vi "Shot Info Collection.vi"(6 "Vision Target Aligned? in":bool, 7 "Current Angle":dbl, 9 "Shot Type":T1, 10 "Vision Packet":T2, 11 "Shooter Presets":T3={"Batter Shot"={"Left"=0.0, "Right"=0.0, "Angle"=0.0}, "Deep Middle Shot"={"Left"=0.0, "Right"=0.0, "Angle"=0.0}, "Manual Shot"={"Left"=0.0, "Right"=0.0, "Angle"=0.0}, "Left Ticks Per Rotation"=0.0, "Right Ticks Per Rotation"=0.0, "Low Bar Shot"={"Left"=0.0, "Right"=0.0, "Angle"=0.0}, "Shooter RPM Tolerance"=0.0, "IIR Filter Power"=0.0, "Trigger Power"=0.0, "Fire from Load Delay"=0, "Max Angle"=0.0, "Min Angle"=0.0, "Angle PID gains"={"P"=0.0, "I"=0.0, "D"=0.0}, "Angle Output"={"output high"=0.0, "output low"=0.0}, "Shooter Angle Tolerance"=0.0, "Vision Shoot x^2"=0.0, "Vision Shoot x"=0.0, "Offset Angle"=0.0, "High Goal Center Height"=0.0, "Feed Forward Max Accel"=0.0, "Feed Forward Kv"=0.0, "Backwards Trigger"=0.0, "Shot Finish Delay (ms)"=0.0, "Angle Max Current"=0.0, "Angle Current Trip Time"=0.0, "Intake Angle"=0.0, "Vision Shoot c"=0.0, "Reset?"=FALSE, "Servo Release Delay"=0.0, "Servo Idle Angle"=0, "Servo Hold Angle"=0, "Angle Pot x"=0.0, "Angle Pot c"=0.0, "Ignore Angle?"=FALSE, "Manual Output?"=FALSE, "Manual Out"=0.0, "Max RPM"=0.0, "Safty Frist Angle"=0.0, "Intake Danger Height"=0.0, "Angle Pot B"=0, "Angle Pot M"=0.0, "FF Finish RPM"=0.0, "RPM PID Right"={"P"=1.0, "I"=0.01, "D"=0.0, "FF"=0.0}, "RPM PID Left"={"P"=1.0, "I"=0.01, "D"=0.0, "FF"=0.0}, "Backwards RPM"=0.0, "Vision RPM"=0.0, "Run Wheels Backward Delay"=0} {"Angle Output"."output low" format="%.2f"; "Angle Output"."output high" format="%.2f"}) -> (2 "Right Wheel RPM":dbl, 3 "Left Wheel RPM":dbl, 4 "Angle":dbl, 5 "Vision Target Aligned? out":bool)   [LabVIEW 2015]
uses:
  Common Code/Shooter Presets.ctl
  Common Code/Shot Presets.ctl
  Common Code/Goal Vision Packet.ctl
  Common Code/Shot Type.ctl
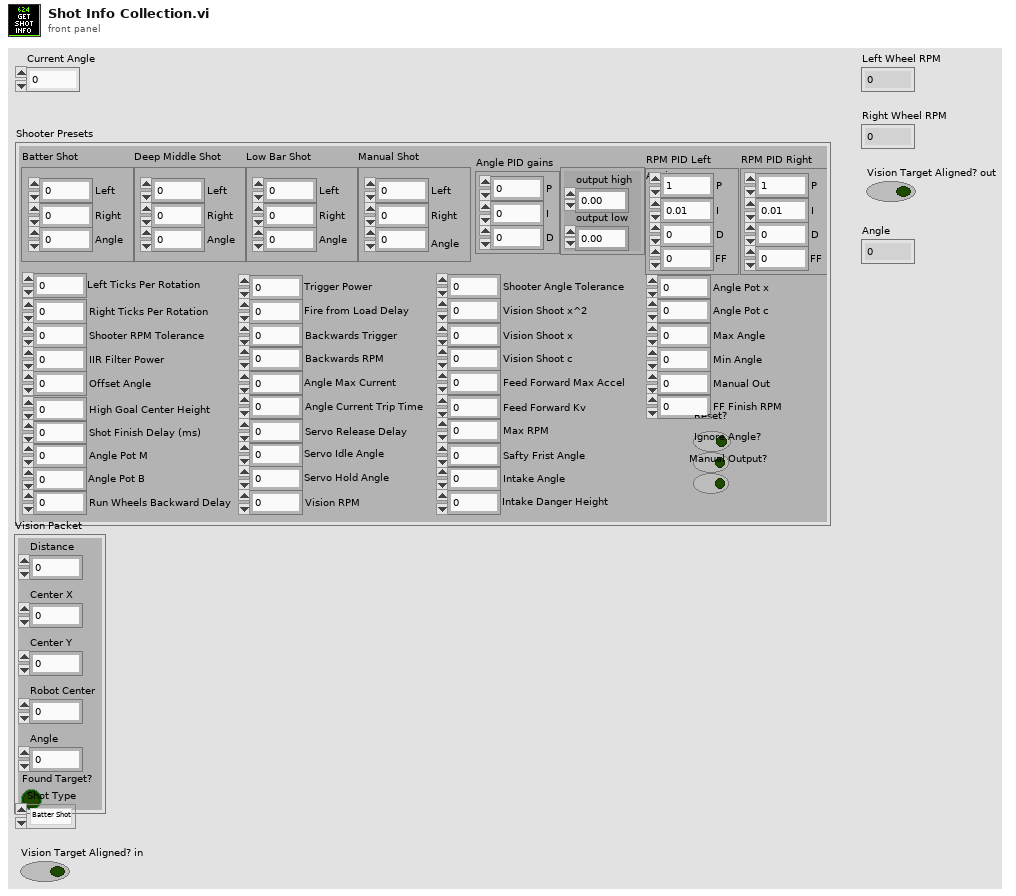
[diagram p1: front panel]
types:
  T1 = typedef "Shot Type.ctl" = enum16{"Batter Shot", "Corner Shot", "Curve Shot", "Vision Shot", "Deep Middle Shot"}
  T2 = typedef "Goal Vision Packet.ctl" = cluster{"Distance":dbl, "Center X":dbl, "Center Y":dbl, "Found Target?":bool, "Robot Center":dbl, "Angle":dbl}
  T3 = typedef "Shooter Presets.ctl" = cluster{"Batter Shot":T4, "Deep Middle Shot":T4, "Manual Shot":T4, "Left Ticks Per Rotation":dbl, "Right Ticks Per Rotation":dbl, "Low Bar Shot":T4, "Shooter RPM Tolerance":dbl, "IIR Filter Power":dbl, "Trigger Power":dbl, "Fire from Load Delay":i32, "Max Angle":dbl, "Min Angle":dbl, "Angle PID gains":cluster{"P":dbl, "I":dbl, "D":dbl}, "Angle Output":cluster{"output high":dbl, "output low":dbl}, "Shooter Angle Tolerance":dbl, "Vision Shoot x^2":dbl, "Vision Shoot x":dbl, "Offset Angle":dbl, "High Goal Center Height":dbl, "Feed Forward Max Accel":dbl, "Feed Forward Kv":dbl, "Backwards Trigger":dbl, "Shot Finish Delay (ms)":dbl, "Angle Max Current":dbl, "Angle Current Trip Time":dbl, "Intake Angle":dbl, "Vision Shoot c":dbl, "Reset?":bool, "Servo Release Delay":dbl, "Servo Idle Angle":i32, "Servo Hold Angle":i32, "Angle Pot x":dbl, "Angle Pot c":dbl, "Ignore Angle?":bool, "Manual Output?":bool, "Manual Out":dbl, "Max RPM":dbl, "Safty Frist Angle":dbl, "Intake Danger Height":dbl, "Angle Pot B":i32, "Angle Pot M":dbl, "FF Finish RPM":dbl, "RPM PID Right":cluster{"P":dbl, "I":dbl, "D":dbl, "FF":dbl}, "RPM PID Left":cluster{"P":dbl, "I":dbl, "D":dbl, "FF":dbl}, "Backwards RPM":dbl, "Vision RPM":dbl, "Run Wheels Backward Delay":u32}
  T4 = typedef "Shot Presets.ctl" = cluster{"Left":dbl, "Right":dbl, "Angle":dbl}
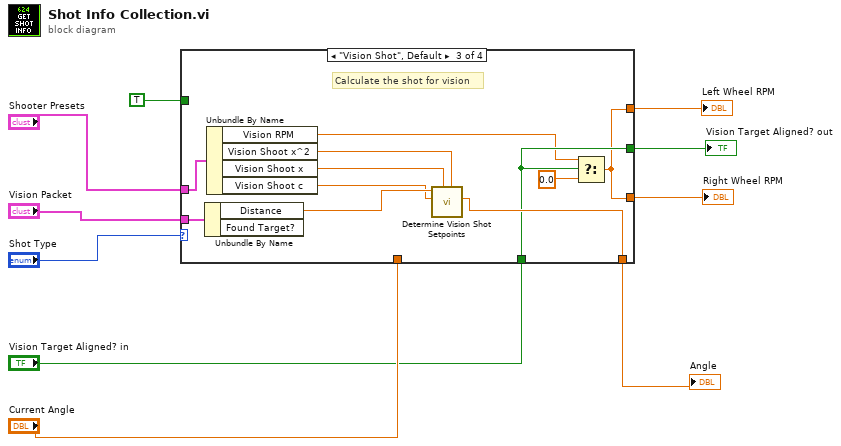
[diagram p0: block diagram]
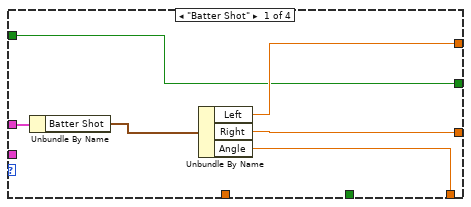
[diagram p2: hidden frame]
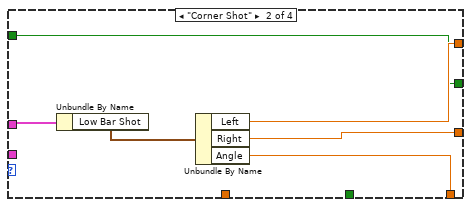
[diagram p3: hidden frame]
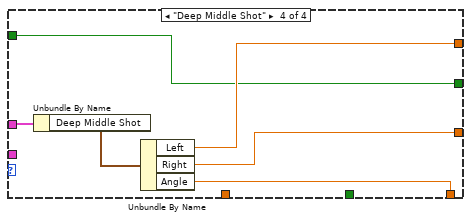
[diagram p4: hidden frame]
diagram:
  n1 = case shown="\"Vision Shot\", Default" "Shot Type" {
    tunnel: "Shooter Presets" -> [w16 w22 w33 w39]
    tunnel: [w14 w18 w23 w37] -> w2
    tunnel: [w13 w19 w23 w36] -> w3
    tunnel: "Vision Packet" -> [_ _ w31 _]
    tunnel: [w12 w17 w26 w35] -> w5
    tunnel: "Vision Target Aligned? in" -> [_ _ w26 _]
    tunnel: TRUE -> [w12 w17 _ w35]
    tunnel: [w11 w20 w30 w34] -> w8
    tunnel: "Current Angle" -> [_ _ _ _]
    frame "Batter Shot" {
      n2 = Unbundle By Name(w16) -> ("Batter Shot"=w15:T4)
      n3 = Unbundle By Name(w15) -> ("Left"=w14:dbl, "Right"=w13:dbl, "Angle"=w11:dbl)
    }
    frame "Corner Shot" {
      n4 = Unbundle By Name(w22) -> ("Low Bar Shot"=w21:T4)
      n5 = Unbundle By Name(w21) -> ("Left"=w18:dbl, "Right"=w19:dbl, "Angle"=w20:dbl)
    }
    frame "Vision Shot", Default {
      # "Calculate the shot for vision"
      n6 = Unbundle By Name(w31) -> ("Distance"=w32:dbl)  [unwired: 1 out]
      n7 = Unbundle By Name(w33) -> ("Vision RPM"=w25:dbl, "Vision Shoot x^2"=w28:dbl, "Vision Shoot x"=w29:dbl, "Vision Shoot c"=w27:dbl)
      n8 = call "Determine Vision Shot Setpoints.vi"("x^2"=w28, "x"=w29, "c"=w27, "Distance from Target"=w32) -> ("Angle"=w30:dbl)  [unwired: 7 in]
      n9 = Select(t=w25, s=w26, f=0.0) -> (s? t:f=w23:dbl)
    }
    frame "Deep Middle Shot" {
      n10 = Unbundle By Name(w39) -> ("Deep Middle Shot"=w38:T4)
      n11 = Unbundle By Name(w38) -> ("Left"=w37:dbl, "Right"=w36:dbl, "Angle"=w34:dbl)
    }
  }
  "Angle" <- w8
  "Vision Target Aligned? out" <- w5
  "Right Wheel RPM" <- w3
  "Left Wheel RPM" <- w2
